vi "GUI_laptop v11b.vi"() -> ()   [LabVIEW 2019]
uses:
  <vilib>/Math Plots/3D Math Plots/3D Scatter/3D Scatter XCtrl/3D Scatter.xctl
  <vilib>/Platform/TimedLoop/XDataNode/timing_clust.ctl
  <vilib>/Platform/TimedLoop/XDataNode/nitl_modes.ctl
  <vilib>/Platform/TimedLoop/XDataNode/wakeup.ctl
  <vilib>/Analysis/_algsub.llb/Real Vector Norm.vi
  <vilib>/Instr/_visa.llb/VISA Configure Serial Port (Instr).vi
  <vilib>/Utility/file.llb/Write Delimited Spreadsheet (DBL).vi
  <vilib>/Math Plots/3D Math Plots/3D Scatter/3D Scatter Datatype/Public/Plot Helper (Vector).vi
  <vilib>/platform/TimedLoop/XDataNode/XDataNode.xnode
  <vilib>/Platform/TimedLoop/XDataNode/XDNodeRunTimeDep.lvlib
  <vilib>/Analysis/NI_AALPro.lvlib
  <vilib>/Math Plots/3D Math Plots/3D Scatter/3D Scatter Datatype/3D Scatter Datatype.lvclass
panel:
  out "spreadsheet string":string
  out "1-D Array of Real 2":dbl[](array[numeric])
  out "1-D Array of Real":dbl[](array[numeric])
  in  "Save Path 2":path=path "C:/Users/jimmy/Documents/GitHub/Arduino-LabVIEW/zhantao/read_data_delt.csv"
  out "Numeric":i32
  out "send values":dbl[](array[numeric])
  out "Robot Feedback (xyz)":dbl[](array[numeric])
  in  "UDP Send":bool
  in  "UDP Recv":bool
  in  "L5 bound":dbl=1000.0
  in  "L4 bound (deg)":dbl=1000.0
  in  "L3 bound (mm)":dbl=1000.0
  in  "L2 bound (deg)":dbl=1000.0
  in  "L1 bound (deg)":dbl=1000.0
  in  "Joystick Type":dbl(ring) items=["Rigid Joystick", "Free Joystick"]
  out "Finished Late? [i-1]":bool
  in  "Epsilon":dbl=0.2
  out "3D Scatter":refnum<class "3D Plot Datatype.lvclass">[](xcontrol)
  out "Random Point":dbl[](array[numeric])
  out "Virtual Cursor":dbl[](array[numeric])
  out "Iteration Duration":i64
  in  "Num of Points":i32=10
  in  "z bound":dbl=2.0
  in  "y bound":dbl=5.0
  in  "x bound":dbl=5.0
  in  "Stop":bool
  in  "Round Decimals":dbl=2.0 format="%#_15g"
  in  "Save  Data":bool
  in  "Save Path":path=path "C:/Users/jimmy/Documents/GitHub/Arduino-LabVIEW/zhantao/read_data_abs.csv"
  in  "x speed":dbl=0.5
  in  "z speed":dbl=0.5
  in  "y speed":dbl=0.5
  out "error out":errorcluster
  in  "baud rate":u32=115200
  in  "VISA resource name":refnum<visa-resource-name>
  # "TODO: fix the bounds; currently bounds are arbitrary"
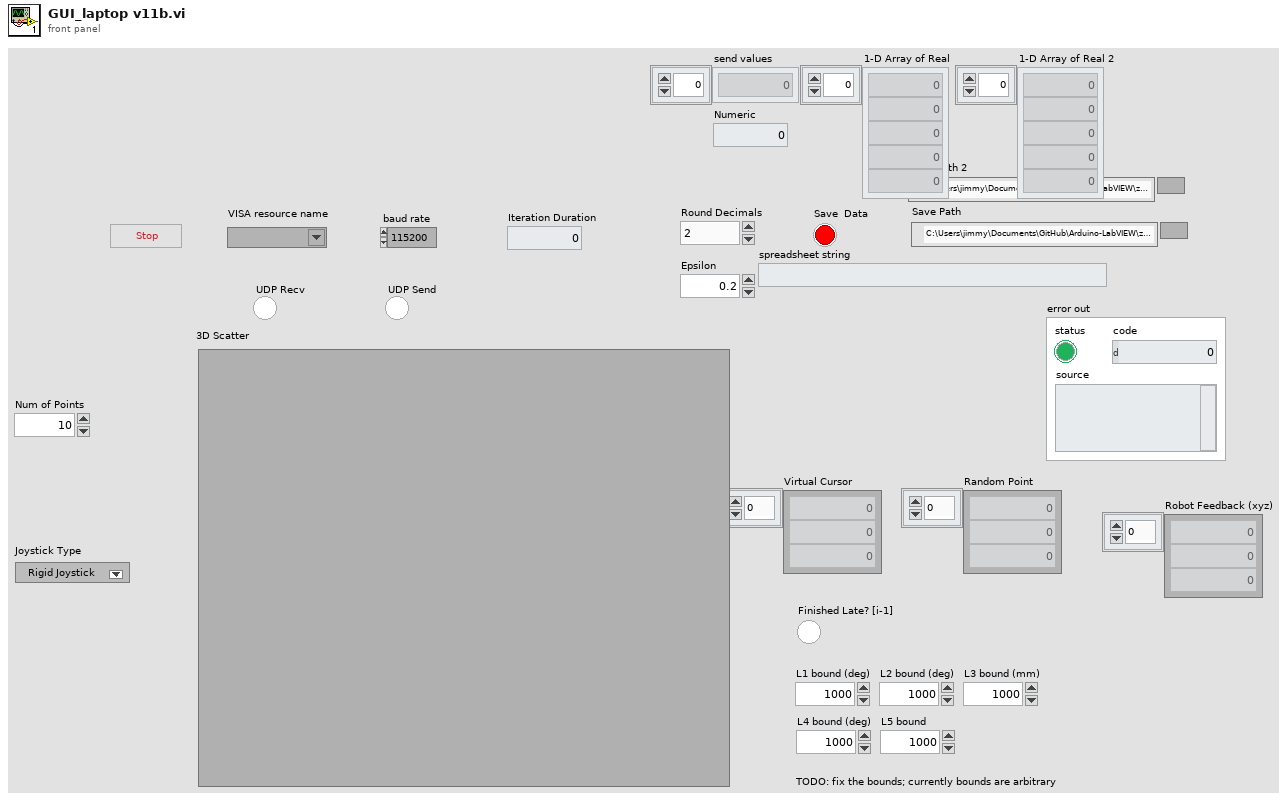
[diagram p1: front panel]
types:
  T1 = typedef "XDNodeRunTimeDep.lvlib/timing_clust.ctl" = cluster{"Expected End [f-1]":u64, "Actual End [f-1]":u64, "Finished Late? [f-1]":bool, "Expected End [i-1]":u64, "Actual End [i-1]":u64, "Finished Late? [i-1]":bool, "Expected Start [i]":u64, "Actual Start [i]":u64, "Expected Start [f]":u64, "Actual Start [f]":u64, "Source Name":string, "Structure Name":string, "Period":i64, "Deadline":i64, "Offset":i64, "Start":i64, "Priority":i32, "Timeout":i32, "Mode":T2, "Wakeup Reason":T3, "Error":errorcluster, "Source Type":string, "Secondary Source Type":string, "Global End Time":u64, "Global Start Time":u64, "Frame Duration":u64, "Iteration Duration":u64, "Assigned CPU":i32, "I/O Scan Engine Mode":u32}
  T2 = typedef "XDNodeRunTimeDep.lvlib/nitl_modes.ctl" = enum32{"No Change", "Process missed periods, maintain original phase", "Discard missed periods, maintain original phase", "Process missed periods, ignore original phase", "Discard missed periods, ignore original phase"}
  T3 = typedef "XDNodeRunTimeDep.lvlib/wakeup.ctl" = enum32{"Normal", "Aborted", "Asynchronous wakeup", "Timing source error", "Timed loop error", "Timeout"}
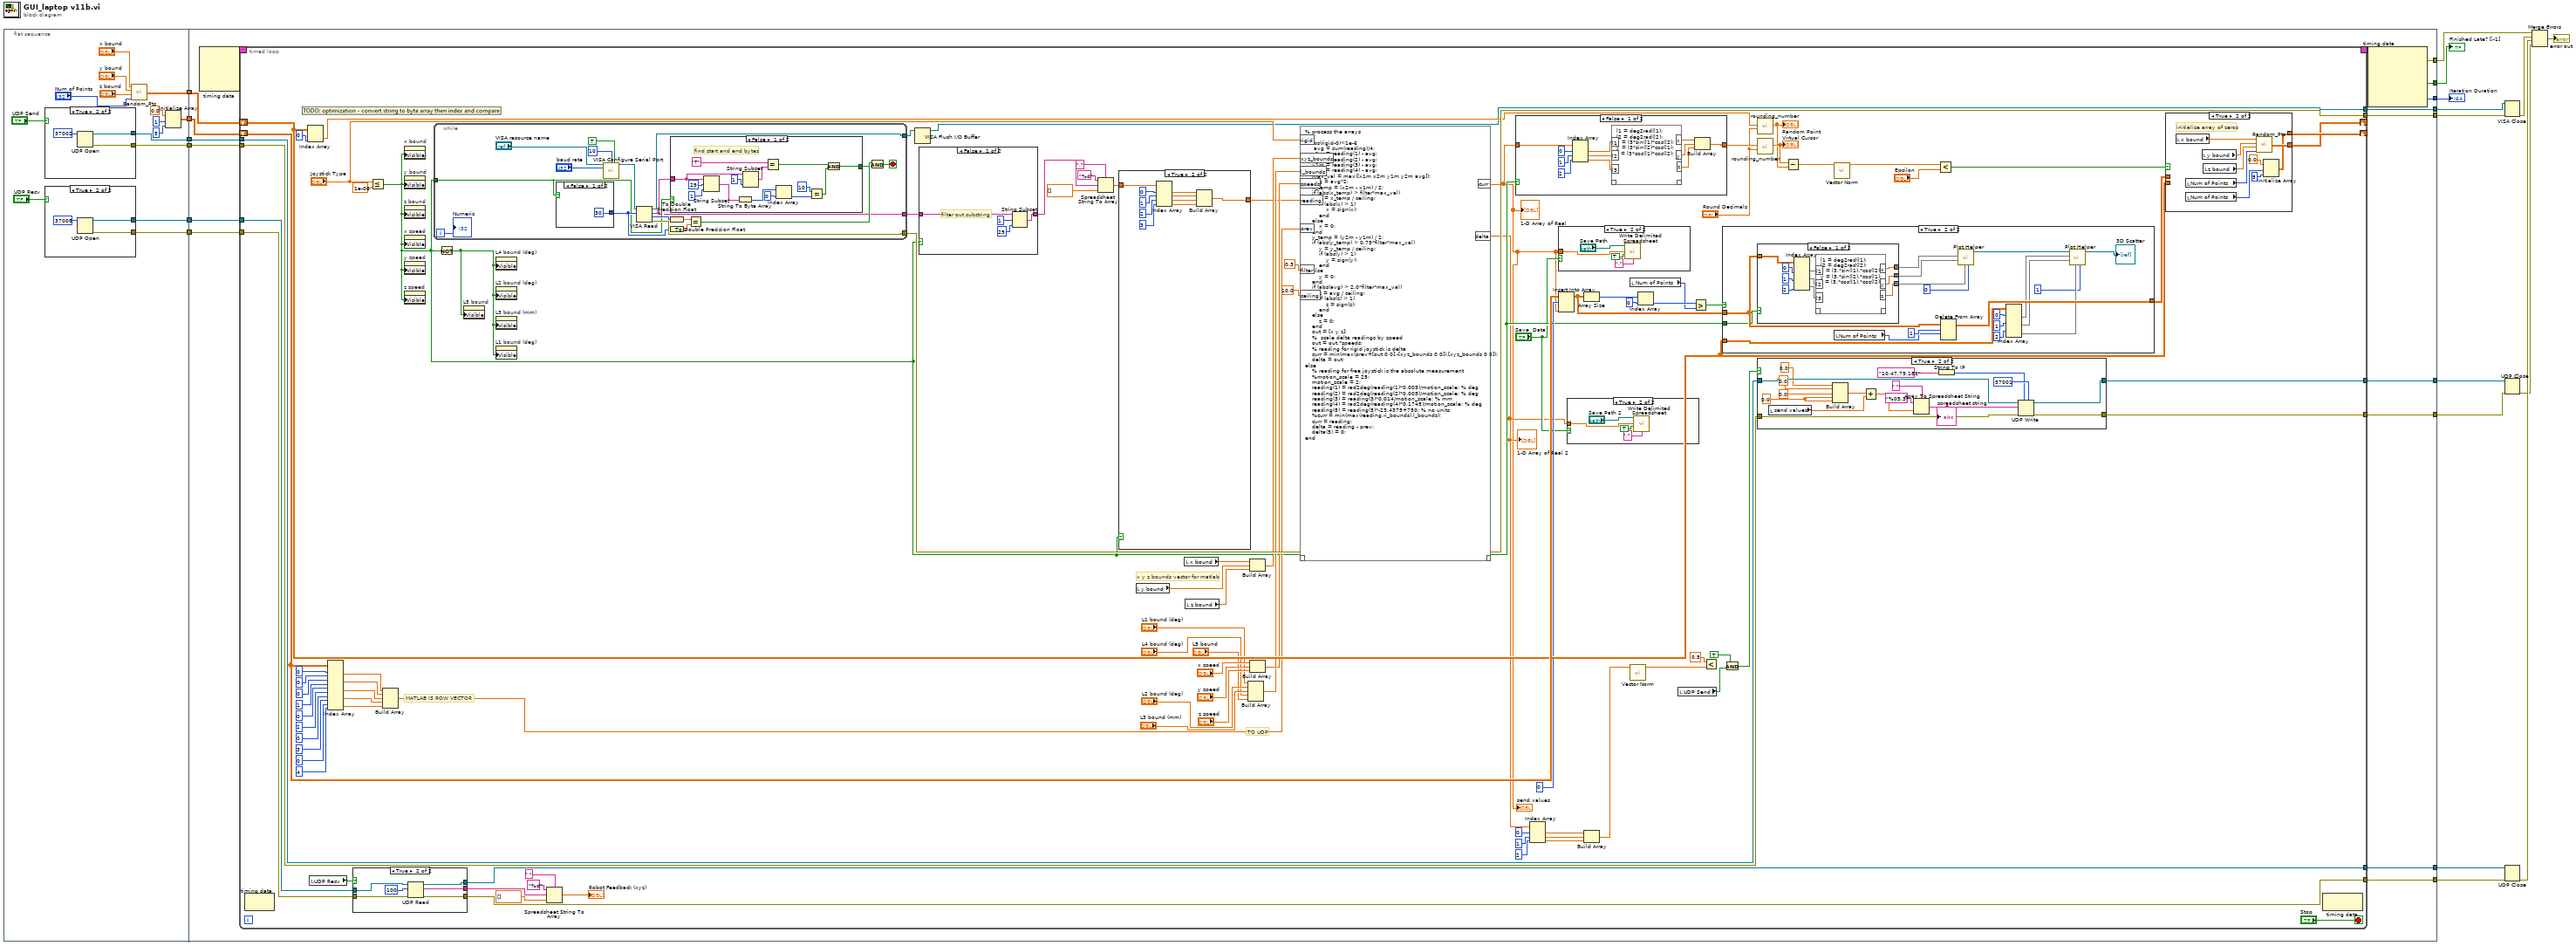
[diagram p0: block diagram]
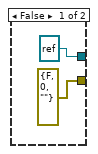
[diagram p2: hidden frame]
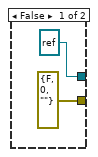
[diagram p3: hidden frame]
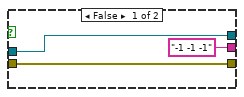
[diagram p6: hidden frame]
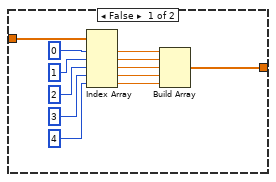
[diagram p10: hidden frame]
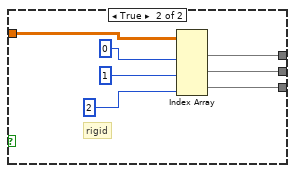
[diagram p13: hidden frame]
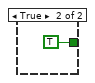
[diagram p14: hidden frame]
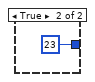
[diagram p15: hidden frame]
diagram:
  n1 = flat-sequence {
    tunnel: [w26] -> w15
    tunnel: [w30] -> w14
    tunnel: [w25] -> w13
    tunnel: [w24] -> w12
    tunnel: [w21] -> w11
    tunnel: [w20] -> w10
    tunnel: [w59] -> w19
    tunnel: [w58] -> w18
    tunnel: [w56] -> w9
    tunnel: [w54] -> w17
    tunnel: [w53] -> w16
    tunnel: w15 -> [w57]
    tunnel: w14 -> [w55]
    tunnel: w13 -> [w52]
    tunnel: w12 -> [w51]
    tunnel: w11 -> [w50]
    tunnel: w10 -> [w49]
    tunnel: [w48] -> w3
    tunnel: [w47] -> w8
    tunnel: [w46] -> w2
    tunnel: [w45] -> w1
    frame #0 {
      n2 = case shown="True" "UDP Send" {
        tunnel: [refnum<k16> refnum ("port") w38] -> w25
        tunnel: [errorcluster {"status"=FALSE, "code"=0, "source"=""} ("error out") w37] -> w20
        frame False {
        }
        frame True {
          n3 = UDP Open(11:u16 37002 ("port")) -> (port=w38:refnum<k16>, 0:w37:errorcluster)  [unwired: 4 in, 1 out]
        }
      }
      n4 = case shown="True" "UDP Recv" {
        tunnel: [refnum<k16> refnum ("port") w43] -> w24
        tunnel: [errorcluster {"status"=FALSE, "code"=0, "source"=""} ("error out") w42] -> w21
        frame False {
        }
        frame True {
          n5 = UDP Open(11:u16 37008 ("port")) -> (port=w43:refnum<k16>, 0:w42:errorcluster)  [unwired: 4 in, 1 out]
        }
      }
      n6 = call "Random_Pts.vi"("Num of Points"="Num of Points", "z bound"="z bound", "y bound"="y bound", "x bound"="x bound") -> ("appended array"=w30:dbl[][])
      n7 = Initialize Array(0.0 ("element"), 1 ("dimension size"), 5 ("dimension size")) -> (w26:dbl[][])
    }
    frame #1 {
      n8 = node-c288() -> (w61:T1)  [unwired: 4 in]
      n9 = timed-loop {
        tunnel: [w66] -> w59
        tunnel: [w158] -> w58
        shift-right: [w157] -> _
        shift-left: w57 -> [w156]
        timing: w61 -> [_]
        timing-out: [_] -> w60
        shift-right: [w152] -> _
        shift-left: w55 -> [w153]
        tunnel: w52 -> [w96]
        tunnel: w51 -> [w95]
        tunnel: w50 -> [w93]
        tunnel: w49 -> [w92]
        tunnel: [w91] -> w48
        tunnel: [w90] -> w47
        tunnel: [w89] -> w46
        tunnel: [w88] -> w45
        stop <- "Stop" stop-if-true
        # "TO UDP"
        # "MATLAB IS ROW VECTOR"
        # "x y z bounds vector for matlab"
        n10 = node-c288() -> ()  [unwired: 1 in, 1 out]
        n11 = Index Array(array=w153, index (col)=0 ("index (row)")) -> (element=w105:dbl[])  [unwired: 1 in]
        n12 = local read "UDP Recv"() -> (w94:bool)
        n13 = Index Array(array=w156, index (row) #1=0 ("disabled index (row)"), index (col) #1=0 ("disabled index (col)"), index (row) #2=0 ("disabled index (row)"), index (col) #2=1 ("disabled index (col)"), index (row) #3=0 ("disabled index (row)"), index (col) #3=2 ("disabled index (col)"), index (row) #4=0 ("disabled index (row)"), index (col) #4=3 ("disabled index (col)"), index (row) #5=0 ("disabled index (row)"), index (col) #5=4 ("disabled index (col)")) -> (element #1=w129:dbl, element #2=w128:dbl, element #3=w127:dbl, element #4=w113:dbl, element #5=w112:dbl)
        n14 = case shown="True" w94 {
          tunnel: w95 -> [w184 w191]
          tunnel: w93 -> [w185 w190]
          tunnel: [w185 w189] -> w91
          tunnel: [w184 w188] -> w89
          tunnel: ["-1 -1 -1" w186] -> w84
          frame False {
          }
          frame True {
            n15 = UDP Read(connection ID=w191, max size (548)=100, 8:w190) -> (data out=w186:string, error out=w189:errorcluster, 3:w188:refnum<k16>)  [unwired: 1 in, 2 out]
          }
        }
        n16 = Less Or Equal?(x="Joystick Type", y=1e-06) -> (x <= y?=w71:bool)
        n17 = Build Array(w129, w128, w127, w113, w112) -> (w126:dbl[])
        n18 = property on="x bound" class="DigNum (strict)"("Visible"=w71) -> ()  [unwired: 2 in, 2 out]
        n19 = property on="y bound" class="DigNum (strict)"("Visible"=w71) -> ()  [unwired: 2 in, 2 out]
        n20 = property on="z bound" class="DigNum (strict)"("Visible"=w71) -> ()  [unwired: 2 in, 2 out]
        n21 = property on="x speed" class="DigNum (strict)"("Visible"=w71) -> ()  [unwired: 2 in, 2 out]
        n22 = property on="y speed" class="DigNum (strict)"("Visible"=w71) -> ()  [unwired: 2 in, 2 out]
        n23 = property on="z speed" class="DigNum (strict)"("Visible"=w71) -> ()  [unwired: 2 in, 2 out]
        n24 = while {
          tunnel: [w284] -> w107
          tunnel: [w297] -> w158
          tunnel: [w291] -> w67
          tunnel: w71 -> [w285]
          i -> [w283]
          stop <- w287 stop-if-true
          n25 = case shown="False" w285 {
            tunnel: [30 u32 23 ("byte count")] -> w290
            frame False {
            }
            frame True {
            }
          }
          n26 = call-poly "VISA Configure Serial Port"("VISA resource name"="VISA resource name", "termination char\n(0xA = '\\n' = LF)"=u8 10 ("termination char\n(0xA = '\\n' = LF)"), "Enable Termination\nChar (T)"=TRUE ("Enable Termination\nChar (T)"), "baud rate (9600)"="baud rate") -> ("VISA resource name out"=w292:refnum<visa-resource-name>)  [unwired: 10 in, 1 out]
          n27 = VISA Read(VISA resource name=w292, byte count=w290) -> (VISA resource name out=w291:refnum<visa-resource-name>, read buffer=w284:string, return count=w299:u32, error out=w297:errorcluster)  [unwired: 1 in]
          n28 = To Double Precision Float(number=w299) -> (double precision float=w298:dbl)
          n29 = To Double Precision Float(number=w290) -> (double precision float=w289:dbl)
          n30 = case shown="False" w285 {
            tunnel: [w306 TRUE] -> w286
            tunnel: w284 -> [w309 _]
            frame False {
              # "find start and end bytes"
              n31 = String Subset(string=w309, offset (0)=29, length (rest)=1) -> (substring=w304:string)
              n32 = String To Byte Array(string=w304) -> (unsigned byte array=w303:u8[])
              n33 = String Subset(string=w309, length (rest)=1) -> (substring=w312:string)  [unwired: 1 in]
              n34 = Equal?(x="T", y=w312) -> (x = y?=w308:bool)
              n35 = Index Array(array=w303, index=0) -> (element=w301:u8)
              n36 = Equal?(x=10, y=w301) -> (x = y?=w307:bool)
              n37 = And(x=w308, y=w307) -> (x .and. y?=w306:bool)
            }
            frame True {
            }
          }
          n38 = Equal?(x=w298, y=w289) -> (x = y?=w288:bool)
          n39 = And(x=w288, y=w286) -> (x .and. y?=w287:bool)
          "Numeric" <- w283
        }
        n40 = Not(x=w71) -> (.not. x?=w70:bool)
        n41 = property on="L5 bound" class="DigNum (strict)"("Visible"=w70) -> ()  [unwired: 2 in, 2 out]
        n42 = property on="L4 bound (deg)" class="DigNum (strict)"("Visible"=w70) -> ()  [unwired: 2 in, 2 out]
        n43 = property on="L2 bound (deg)" class="DigNum (strict)"("Visible"=w70) -> ()  [unwired: 2 in, 2 out]
        n44 = property on="L3 bound (mm)" class="DigNum (strict)"("Visible"=w70) -> ()  [unwired: 2 in, 2 out]
        n45 = property on="L1 bound (deg)" class="DigNum (strict)"("Visible"=w70) -> ()  [unwired: 2 in, 2 out]
        n46 = Spreadsheet String To Array(delimiter (Tab)=" ", format string="%d", spreadsheet string=w84, array type (2D Dbl)=dbl[] []) -> (array=→"Robot Feedback (xyz)":dbl[])
        n47 = VISA Flush I/O Buffer(VISA resource name=w67) -> (VISA resource name out=w66:refnum<visa-resource-name>)  [unwired: 2 in, 1 out]
        n48 = case shown="False" w71 {
          tunnel: w107 -> [w210 w211]
          tunnel: [w207 w211] -> w106
          frame False {
            # "filter out substring"
            n49 = String Subset(string=w210, offset (0)=1, length (rest)=29) -> (substring=w207:string)
          }
          frame True {
          }
        }
        n50 = Spreadsheet String To Array(delimiter (Tab)=",", format string="%d", spreadsheet string=w106, array type (2D Dbl)=dbl[] []) -> (array=w109:dbl[])
        n51 = case shown="True" w71 {
          tunnel: w109 -> [w212 w227]
          tunnel: [w217 w226] -> w108
          frame False {
            n52 = Index Array(array=w212, index #1=0 ("Plot ID"), index #2=1 ("Plot ID"), index #3=2 ("Plot ID"), index #4=3 ("Plot ID"), index #5=4 ("Plot ID")) -> (element #1=w220:dbl, element #2=w219:dbl, element #3=w218:dbl, element #4=w214:dbl, element #5=w213:dbl)
            n53 = Build Array(w220, w219, w218, w214, w213) -> (w217:dbl[])
          }
          frame True {
            n54 = Index Array(array=w227, index #1=0 ("Plot ID"), index #2=1 ("Plot ID"), index #3=2 ("Plot ID"), index #4=3 ("index")) -> (element #1=w230:dbl, element #2=w229:dbl, element #3=w228:dbl, element #4=w224:dbl)
            n55 = Build Array(w230, w229, w228, w224) -> (w226:dbl[])
          }
        }
        n56 = local read "y bound"() -> (w131:dbl)
        n57 = local read "x bound"() -> (w132:dbl)
        n58 = local read "z bound"() -> (w130:dbl)
        n59 = Build Array("L1 bound (deg)", "L2 bound (deg)", "L3 bound (mm)", "L4 bound (deg)", "L5 bound") -> (w120:dbl[])
        n60 = Build Array(w132, w131, w130) -> (w124:dbl[])
        n61 = Build Array("x speed", "y speed", "z speed") -> (w125:dbl[])
        n62 = script code="% process the arrays\n\nif abs(rigid-0)<1e-6\n     avg = sum(reading)/4;\n    x1m = reading(1) - avg;\n    x2m = reading(2) - avg;\n    y1m = reading(3) - avg;\n    y2m = reading(4) - avg;\n    max_val = max([x1m x2m y1m y2m avg]);\n    avg = avg*2;\n    x_temp = (x2m - x1m) / 2;\n    if (abs(x_temp) > filter*max_val)\n        x = x_temp / ceiling;\n        if (abs(x) > 1)\n            x = sign(x);\n        end\n    else\n        x = 0;\n    end\n    y_temp = (y2m - y1m) / 2;\n    if (abs(y_temp) > 0.75*filter*max_val)\n        y = y_temp / ceiling;\n        if (abs(y) > 1)\n            y = sign(y);\n        end\n    else\n        y = 0;\n    end\n    if (abs(avg) > 2.0*filter*max_val)\n        z = avg / ceiling;\n        if (abs(z) > 1)\n            z = sign(z);\n        end\n    else\n        z = 0;\n    end\n    out = [x y z];\n    %  scale delta readings by speed\n    out = out.*speeds;\n    % reading for rigid joystick is delta\n    curr = min(max(prev+[out 0 0],-[xyz_bounds 0 0]),[xyz_bounds 0 0]);\n    delta = out;\nelse\n    % reading for free joystick is the absolute measurement\n    %motion_scale = 25;\n    motion_scale = 2;\n    reading(1) = rad2deg(reading(1)*0.005)/motion_scale; % deg\n    reading(2) = rad2deg(reading(2)*0.005)/motion_scale; % deg\n    reading(3) = reading(3)*0.014/motion_scale; % mm\n    reading(4) = rad2deg(reading(4)*0.1745)/motion_scale; % deg\n    reading(5) = reading(5)*-23.4375+750; % no units\n    %curr = min(max(reading,-l_bounds),l_bounds);\n    curr = reading;\n    delta = reading - prev;\n    delta(5) = 0;\nend"("xyz_bounds"=w124, "speeds"=w125, "reading"=w108, "prev"=w126, "rigid"="Joystick Type", "l_bounds"=w120, "filter"=0.3 ("Real"), "ceiling"=10.0 ("Real")) -> ("curr"=w62:dbl[], "delta"=w63:dbl[])  [unwired: 1 in, 1 out]
        "send values" <- w62
        "1-D Array of Real" <- w62
        "1-D Array of Real 2" <- w63
        n63 = case shown="False" w71 {
          tunnel: w62 -> [w241 w245]
          tunnel: [w234 w245] -> w154
          frame False {
            n64 = Index Array(array=w241, index #1=0 ("Plot ID"), index #2=1 ("Plot ID"), index #3=2 ("Plot ID")) -> (element #1=w240:dbl, element #2=w239:dbl, element #3=w238:dbl)
            n65 = script code="l1 = deg2rad(l1);\nl2 = deg2rad(l2);\nx = l3*sin(l1)*cos(l2);\ny = l3*sin(l2)*cos(l1);\nz = l3*cos(l1)*cos(l2);"("l1"=w240, "l2"=w239, "l3"=w238) -> ("x"=w237:dbl, "y"=w236:dbl, "z"=w235:dbl)  [unwired: 1 in, 1 out]
            n66 = Build Array(w237, w236, w235) -> (w234:dbl[])
          }
          frame True {
          }
        }
        n67 = Index Array(array=w63, index #1=0 ("disabled index (col)"), index #2=1 ("disabled index (col)"), index #3=2 ("disabled index (col)")) -> (element #1=w75:dbl, element #2=w74:dbl, element #3=w73:dbl)
        n68 = case shown="True" "Save  Data" {
          tunnel: w62 -> [_ w193]
          frame False {
          }
          frame True {
            n69 = call-poly <vilib>:"Write Delimited Spreadsheet.vi"("file path (dialog if empty)"="Save Path", "1D data"=w193, "append to file? (new file:F)"=TRUE, "delimiter (\\t)"="," ("delimiter (\\t)")) -> ()  [unwired: 10 in, 2 out]
          }
        }
        n70 = Insert Into Array(array=w156, index (row)=0, new element=w62) -> (w137:dbl[][])  [unwired: 1 in]
        n71 = case shown="True" "Save  Data" {
          tunnel: w63 -> [_ w161]
          frame False {
          }
          frame True {
            n72 = call-poly <vilib>:"Write Delimited Spreadsheet.vi"("file path (dialog if empty)"="Save Path 2", "1D data"=w161, "append to file? (new file:F)"=TRUE, "delimiter (\\t)"="," ("delimiter (\\t)")) -> ()  [unwired: 10 in, 2 out]
          }
        }
        n73 = Array Size(array=w137) -> (size(s)=w139:i32[])
        n74 = Build Array(w75, w74, w73) -> (w72:dbl[])
        n75 = local read "Num of Points"() -> (w138:i32)
        n76 = call-poly <vilib>:"Vector Norm.vi"("Input Vector"=w72) -> ("norm"=w82:dbl)  [unwired: 9 in, 1 out]
        n77 = Index Array(array=w139, index=0) -> (element=w140:i32)
        n78 = local read "UDP Send"() -> (w80:bool)
        n79 = Greater?(x=w140, y=w138) -> (0:w136:bool)
        n80 = Less?(x=0.5, y=w82) -> ()  [unwired: 1 out]
        n81 = case shown="True" w136 {
          tunnel: w137 -> [w246 w264]
          tunnel: [w246 w263] -> w155
          tunnel: w153 -> [_ w262]
          tunnel: w71 -> [_ w247]
          frame False {
          }
          frame True {
            n82 = case shown="False" w247 {
              tunnel: w264 -> [w275 w279]
              tunnel: [w266 w278] -> w253
              tunnel: [w267 w277] -> w252
              tunnel: [w268 w276] -> w251
              frame False {
                n83 = Index Array(array=w275, index (col) #1=0 ("Plot ID"), index (col) #2=1 ("Plot ID"), index (col) #3=2 ("Plot ID")) -> (element #1=w271:dbl[], element #2=w270:dbl[], element #3=w269:dbl[])  [unwired: 3 in]
                n84 = script code="l1 = deg2rad(l1);\nl2 = deg2rad(l2);\nx = l3.*sin(l1).*cos(l2);\ny = l3.*sin(l2).*cos(l1);\nz = l3.*cos(l1).*cos(l2);"("l1"=w271, "l2"=w270, "l3"=w269) -> ("x"=w266:dbl[], "y"=w267:dbl[], "z"=w268:dbl[])  [unwired: 1 in, 1 out]
              }
              frame True {
                # "rigid"
                n85 = Index Array(array=w279, index (col) #1=0 ("disabled index (col)"), index (col) #2=1 ("index (col)"), index (col) #3=2 ("index (col)")) -> (element #1=w278:dbl[], element #2=w277:dbl[], element #3=w276:dbl[])  [unwired: 3 in]
              }
            }
            n86 = local read "Num of Points"() -> (w261:i32)
            n87 = Delete From Array(array=w264, length=1, index (row)=w261) -> (array with subset deleted=w263:dbl[][])  [unwired: 1 in, 1 out]
            n88 = call-poly <vilib>:"Plot Helper.vi"("Plot ID"=0, "z vector"=w251, "y vector"=w252, "x vector"=w253) -> ("3D Plot lvclass Array out"=w255:refnum<class "3D Plot Datatype.lvclass">[])  [unwired: 2 in, 5 out]
            n89 = Index Array(array=w262, index (row) #1=0 ("index (row)"), index (row) #2=1 ("index (row)"), index (row) #3=2 ("index (row)")) -> (element #1=w259:dbl[], element #2=w258:dbl[], element #3=w257:dbl[])  [unwired: 3 in]
            n90 = call-poly <vilib>:"Plot Helper.vi"("Plot ID"=1, "z vector"=w257, "y vector"=w258, "x vector"=w259, "3D Plot lvclass Array in"=w255) -> ("3D Plot lvclass Array out"=→"3D Scatter":refnum<class "3D Plot Datatype.lvclass">[])  [unwired: 1 in, 5 out]
          }
        }
        n91 = And(x=TRUE, y=w80) -> (x .and. y?=w79:bool)
        n92 = call "rounding_number.vi"("power of ten"="Round Decimals", "Array"=w105) -> ("rounded"=w102:dbl[])  [unwired: 9 in]
        "Random Point" <- w102
        n93 = call "rounding_number.vi"("power of ten"="Round Decimals", "Array"=w154) -> ("rounded"=w103:dbl[])  [unwired: 9 in]
        "Virtual Cursor" <- w103
        n94 = case shown="True" w79 {
          tunnel: w96 -> [w164 w182]
          tunnel: w92 -> [w165 w178]
          tunnel: [w165 w174] -> w90
          tunnel: [w164 w173] -> w88
          frame False {
          }
          frame True {
            w172 = 0.0 ("element")
            n95 = local read "send values"() -> (w170:dbl[])
            n96 = Build Array(0.0 ("element"), 0.0 ("element"), 0.0 ("element"), w172, w172) -> (w171:dbl[])
            n97 = Add(x=w171, y=w170) -> (x+y=w169:dbl[])
            n98 = Array To Spreadsheet String(delimiter (Tab)=" ", array=w169, 3:"%05.3f" ("format string")) -> (spreadsheet string=w179:string)
            "spreadsheet string" <- w179
            n99 = String To IP(1:"10.47.79.181" ("name")) -> (0:w176:u32)
            n100 = UDP Write(address=w176, port or service name=u16 37001, connection ID=w182, data in=w179, 8:w178) -> (error out=w174:errorcluster, 3:w173:refnum<k16>)  [unwired: 1 in]
          }
        }
        n101 = Subtract(x=w103, y=w102) -> (x-y=w101:dbl[])
        n102 = call-poly <vilib>:"Vector Norm.vi"("Input Vector"=w101) -> ("norm"=w100:dbl)  [unwired: 9 in, 1 out]
        n103 = Less?(x=w100, y="Epsilon") -> (x < y?=w98:bool)
        n104 = case shown="True" w98 {
          tunnel: w153 -> [w197 _]
          tunnel: [w197 w202] -> w152
          tunnel: w155 -> [w196 _]
          tunnel: [w196 w198] -> w157
          frame False {
          }
          frame True {
            # "initialize array of zeros"
            n105 = local read "x bound"() -> (w206:dbl)
            n106 = local read "Num of Points"() -> (w203:i32)
            n107 = local read "Num of Points"() -> (w200:i32)
            n108 = local read "y bound"() -> (w205:dbl)
            n109 = local read "z bound"() -> (w204:dbl)
            n110 = call "Random_Pts.vi"("Num of Points"=w203, "z bound"=w204, "y bound"=w205, "x bound"=w206) -> ("appended array"=w202:dbl[][])
            n111 = Initialize Array(0.0 ("element"), w200, 5 ("dimension size")) -> (w198:dbl[][])
          }
        }
        n112 = node-c288() -> ()  [unwired: 1 in, 1 out]
      }
      n113 = node-c288(w60) -> (w56:errorcluster, w53:bool, w54:i64)  [unwired: 3 out]
    }
  }
  n114 = VISA Close(VISA resource name=w19, error in (no error)=w18) -> (error out=w7:errorcluster)
  n115 = UDP Close(connection ID=w1, 8:w8) -> (error out=w5:errorcluster)  [unwired: 1 out]
  n116 = UDP Close(connection ID=w2, 8:w3) -> (error out=w6:errorcluster)  [unwired: 1 out]
  n117 = Merge Errors(w9, w7, w6, w5) -> (→"error out":errorcluster)
  "Iteration Duration" <- w17
  "Finished Late? [i-1]" <- w16
